vi "robo_stop.vi"(2 "错误输入（无错误）":errorcluster, 3 "输入 2":i32, 4 "输入 1":i32, 5 "VISA资源名称":refnum<visa-resource-name>) -> (0 "错误输出":errorcluster, 1 "VISA资源名称输出":refnum<visa-resource-name>)   [LabVIEW 2017]
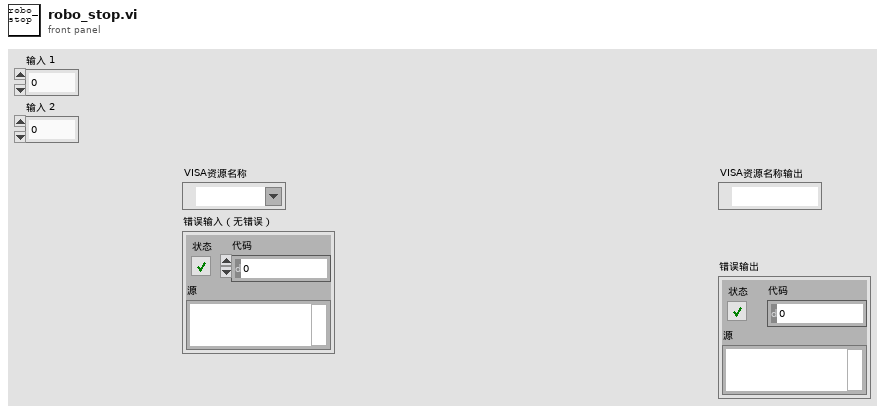
[diagram p1: front panel]
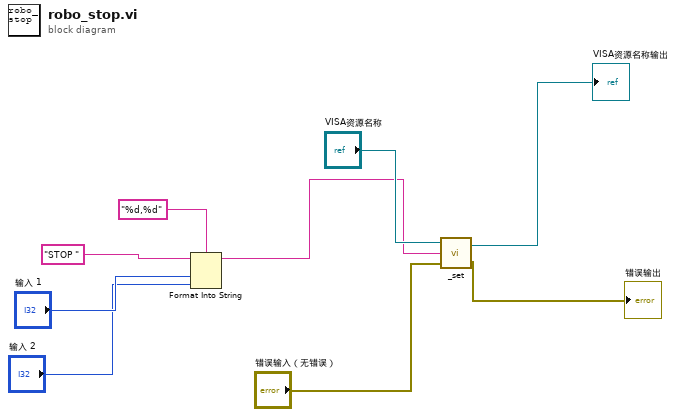
[diagram p0: block diagram]
diagram:
  n1 = Format Into String(format string="%d,%d" ("格式字符串"), initial string="STOP " ("初始字符串"), "输入 1", "输入 2") -> (resulting string=w4:string)  [unwired: 1 in, 1 out]
  n2 = call "_set.vi"("错误输入（无错误）"="错误输入（无错误）", "写入缓冲区"=w4, "连接ID"="VISA资源名称") -> ("错误输出"=→"错误输出":errorcluster, "连接ID输出"=→"VISA资源名称输出":refnum<k5>)
